vi "LS-50.vi"(0 "LS-50 Notifier":refnum<notifier>, 5 "LS-50 Action":T1={"Action"=enum."Get Position", "Axis"=[], "Setpoint"=[], "Velocity"=0.5, "Cmd Recvd?"=FALSE, "Position"=[], "Status"=enum."Error", "Misc"=variant} {"Velocity" min=0.0 max=1.0 step=0.01}, 11 "LS-50 VISA":refnum<visa-resource-name>) -> (4 "LS-50 Notifier (Dup)":refnum<notifier>)   [LabVIEW 2020]
uses:
  Stages Controls/Stage Notifier Element.ctl
  Stages Controls/Stage Actions.ctl
  Stages Controls/Stage Status.ctl
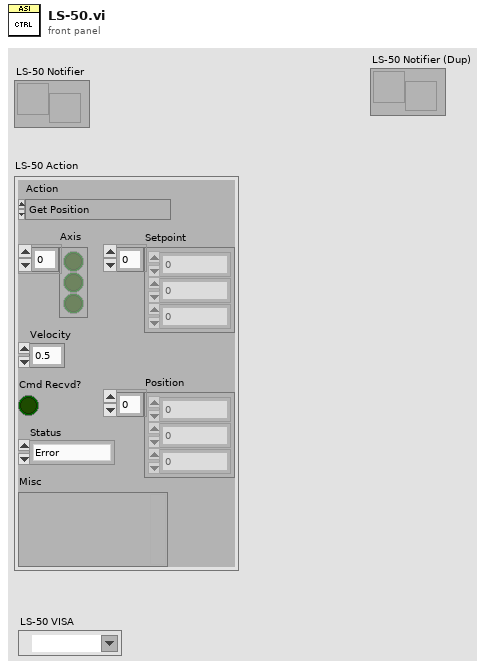
[diagram p1: front panel]
types:
  T1 = typedef "Stage Notifier Element.ctl" = cluster{"Action":T2, "Axis":bool[], "Setpoint":dbl[], "Velocity":dbl, "Cmd Recvd?":bool, "Position":dbl[], "Status":T3, "Misc":variant}
  T2 = typedef "Stage Actions.ctl" = enum16{"Get Position", "MVR", "MOVE", "HALT", "ONTARGET", "ERROR", "REFERENCE", "INIT", "VELOCITY", "STATUS", "EXIT", "HOME", "ZEROPOS", "NANOPOS", "ANALOG", "QUIT"}
  T3 = typedef "Stage Status.ctl" = enum16{"Error", "Abort", "Busy", "On Target"}
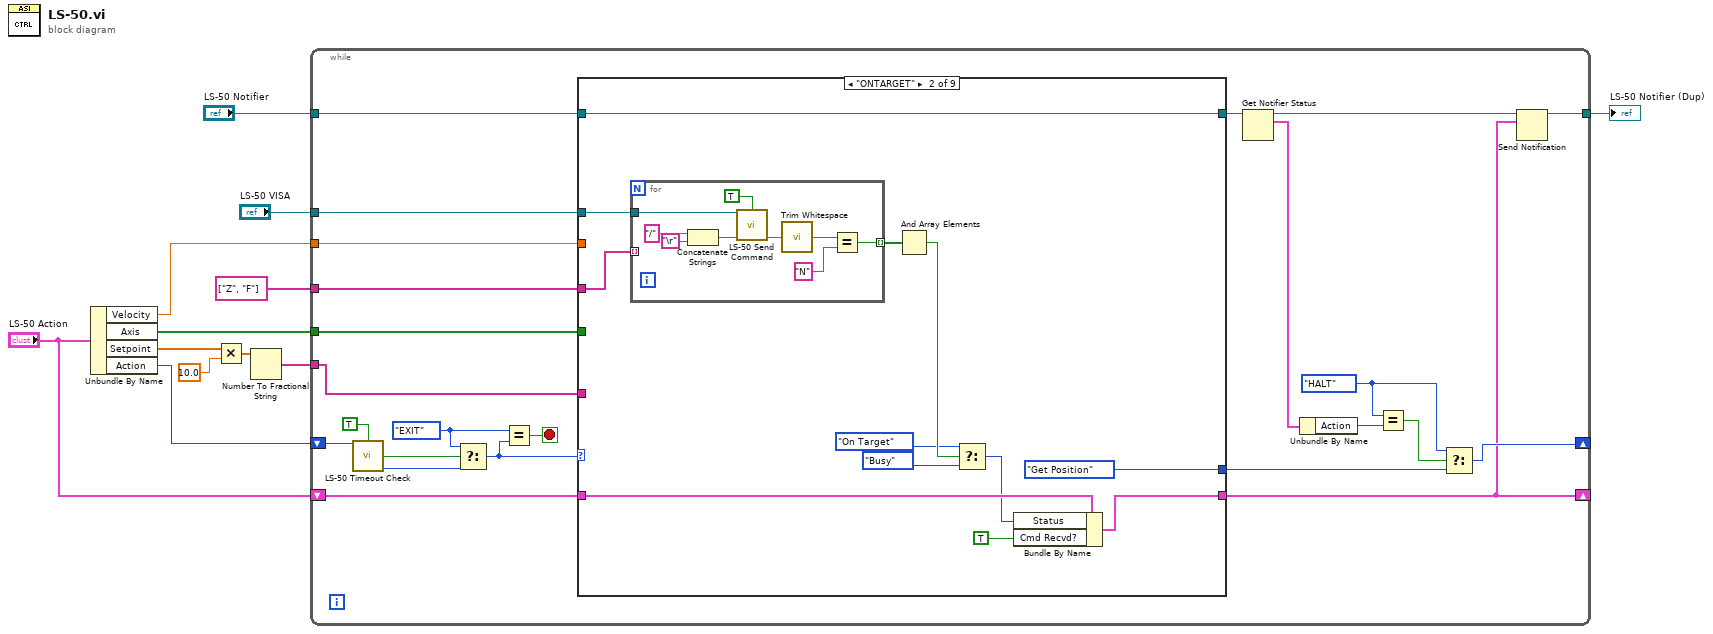
[diagram p0: block diagram]
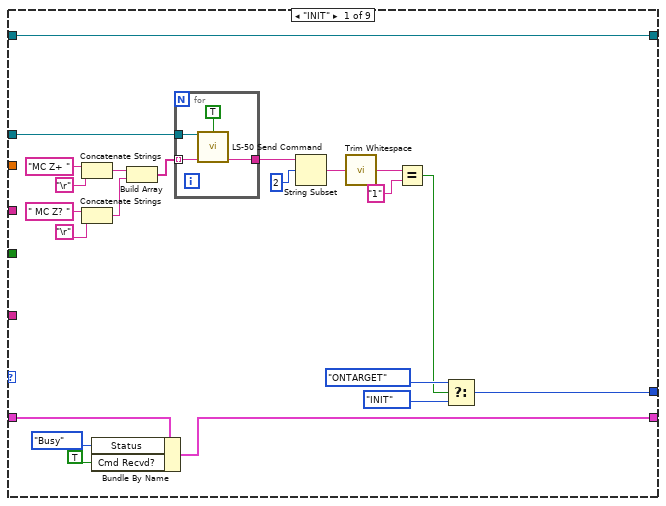
[diagram p2: hidden frame]
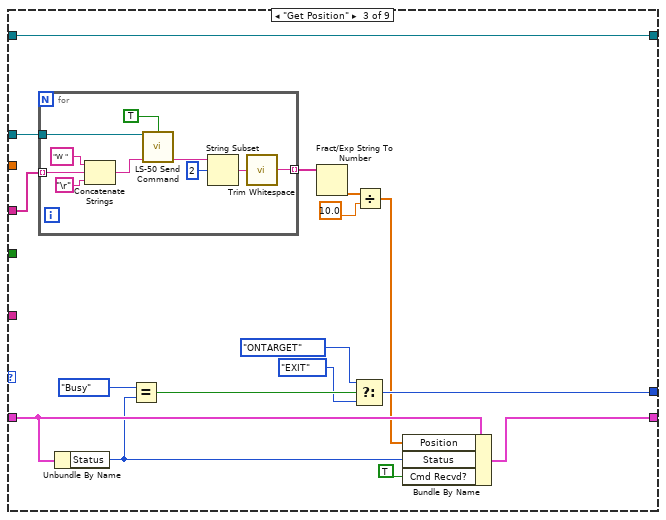
[diagram p3: hidden frame]
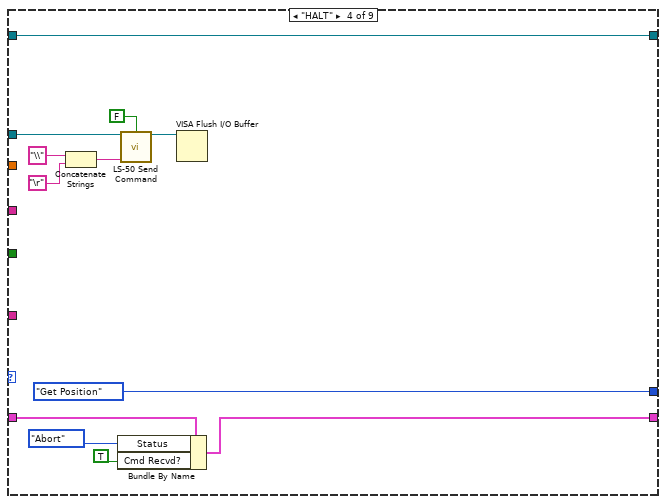
[diagram p4: hidden frame]
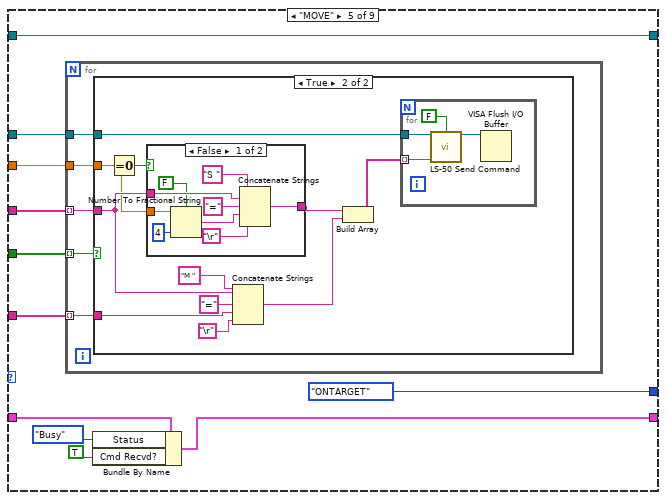
[diagram p5: hidden frame]
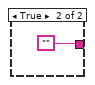
[diagram p7: hidden frame]
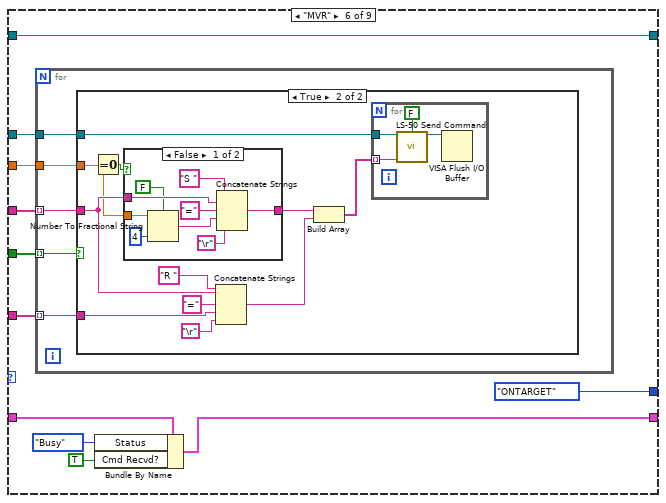
[diagram p8: hidden frame]
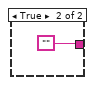
[diagram p10: hidden frame]
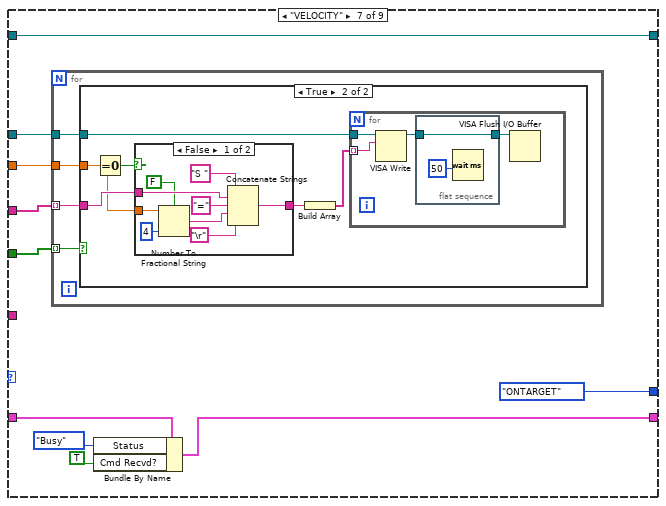
[diagram p11: hidden frame]
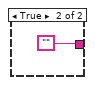
[diagram p13: hidden frame]
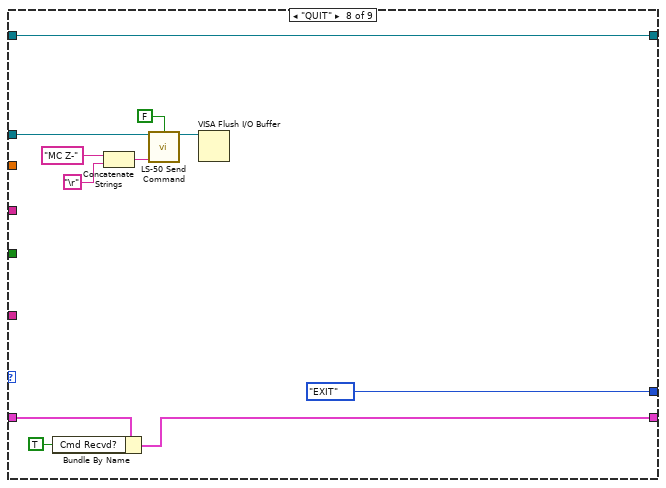
[diagram p14: hidden frame]
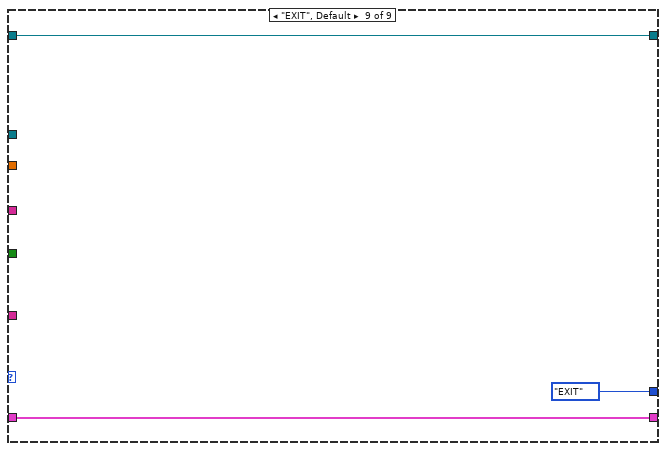
[diagram p15: hidden frame]
diagram:
  n1 = Unbundle By Name("LS-50 Action") -> ("Velocity"=w9:dbl, "Axis"=w8:bool[], "Setpoint"=w5:dbl[], "Action"=w7:T2)
  n2 = Multiply(x=w5, y=10.0) -> (x*y=w6:dbl[])
  n3 = Number To Fractional String(number=w6) -> (F-format string=w10:string[])  [unwired: 3 in]
  n4 = while {
    tunnel: string[] ["Z", "F"] -> [w36]
    shift-right: [w28] -> _
    shift-left: w7 -> [w25]
    tunnel: w8 -> [w33]
    tunnel: w9 -> [w32]
    tunnel: w10 -> [w34]
    shift-right: [w27] -> _
    shift-left: "LS-50 Action" -> [w30]
    tunnel: "LS-50 VISA" -> [w35]
    tunnel: "LS-50 Notifier" -> [w15]
    tunnel: [w13] -> w1
    stop <- w31 stop-if-true
    w17 = Stage_Actions."HALT" ("Action")
    w22 = Stage_Actions."EXIT" ("t")
    n5 = call "LS-50 Timeout Check.vi"("Action"=w25, "User Input?"=TRUE) -> ("Timeout?"=w24:bool, "Action (Dup)"=w23:T2)  [unwired: 12 in]
    n6 = Select(t=w22, s=w24, f=w23) -> (s? t:f=w21:T2)
    n7 = Equal?(x=w22, y=w21) -> (x = y?=w31:bool)
    n8 = case shown="\"ONTARGET\"" w21 {
      tunnel: w36 -> [_ w73 w99 _ w132 w173 w213 _ _]
      tunnel: w35 -> [w40 w64 w85 w114 w123 w164 w205 w244 _]
      tunnel: w34 -> [_ _ _ _ w131 w172 _ _ _]
      tunnel: w33 -> [_ _ _ _ w130 w171 w212 _ _]
      tunnel: w32 -> [_ _ _ _ w129 w170 w211 _ _]
      tunnel: [w50 Stage_Actions."Get Position" ("y") w95 Stage_Actions."Get Position" ("Action") Stage_Actions."ONTARGET" ("y") Stage_Actions."ONTARGET" ("y") Stage_Actions."ONTARGET" ("y") Stage_Actions."EXIT" ("y") Stage_Actions."EXIT" ("y")] -> w29
      tunnel: w30 -> [w47 w70 w90 w116 w128 w166 w207 w246 w253]
      tunnel: [w46 w71 w89 w117 w125 w167 w208 w245 w253] -> w27
      tunnel: [w37 w63 w84 w110 w122 w163 w204 w240 w251] -> w14
      tunnel: w15 -> [w37 w63 w84 w110 w122 w163 w204 w240 w251]
      frame "INIT" {
        n9 = Concatenate Strings("MC Z+ " ("string"), "\r") -> (w43:string)
        n10 = Concatenate Strings(" MC Z? " ("string"), "\r") -> (w42:string)
        n11 = Bundle By Name(cluster=w47, "Status"=Stage_Status."Busy", "Cmd Recvd?"=TRUE) -> (w46:T1)
        n12 = Build Array(w43, w42) -> (w41:string[])
        n13 = for {
          tunnel: [w60] -> w39
          tunnel: w41 -> [w61] mode=indexing
          tunnel: w40 -> [w62]
          n14 = call "LS-50 Send Command.vi"("VISA Ref"=w62, "Read Reply?"=TRUE, "Command"=w61) -> ("Response"=w60:string)  [unwired: 10 in, 2 out]
        }
        n15 = String Subset(string=w39, offset (0)=2) -> (substring=w56:string)  [unwired: 1 in]
        n16 = call <vilib>:"Trim Whitespace.vi"("string"=w56) -> ("trimmed string"=w57:string)  [unwired: 1 in]
        n17 = Equal?(x=w57, y="1") -> (x = y?=w38:bool)
        n18 = Select(t=Stage_Actions."ONTARGET" ("y"), s=w38, f=Stage_Actions."INIT" ("y")) -> (s? t:f=w50:T2)
      }
      frame "ONTARGET" {
        n19 = for {
          tunnel: [w83] -> w74 mode=indexing
          tunnel: w73 -> [_] mode=indexing
          tunnel: w64 -> [w78]
          n20 = Concatenate Strings("/" ("string"), "\r") -> (w77:string)
          n21 = call "LS-50 Send Command.vi"("VISA Ref"=w78, "Read Reply?"=TRUE ("Wait for Reply?"), "Command"=w77) -> ("Response"=w76:string)  [unwired: 10 in, 2 out]
          n22 = call <vilib>:"Trim Whitespace.vi"("string"=w76) -> ("trimmed string"=w80:string)  [unwired: 1 in]
          n23 = Equal?(x=w80, y="N") -> (x = y?=w83:bool)
        }
        n24 = And Array Elements(Boolean array=w74) -> (logical AND=w68:bool)
        n25 = Select(t=Stage_Status."On Target" ("Status"), s=w68, f=Stage_Status."Busy" ("Status")) -> (s? t:f=w66:T3)
        n26 = Bundle By Name(cluster=w70, "Status"=w66, "Cmd Recvd?"=TRUE) -> (w71:T1)
      }
      frame "Get Position" {
        n27 = for {
          tunnel: [w109] -> w98 mode=indexing
          tunnel: w99 -> [w104] mode=indexing
          tunnel: w85 -> [w103]
          n28 = Concatenate Strings("W " ("string"), w104, "\r") -> (w102:string)
          n29 = call "LS-50 Send Command.vi"("VISA Ref"=w103, "Read Reply?"=TRUE ("Wait for Reply?"), "Command"=w102) -> ("Response"=w101:string)  [unwired: 10 in, 2 out]
          n30 = String Subset(string=w101, offset (0)=2) -> (substring=w105:string)  [unwired: 1 in]
          n31 = call <vilib>:"Trim Whitespace.vi"("string"=w105) -> ("trimmed string"=w109:string)  [unwired: 1 in]
        }
        n32 = Unbundle By Name(w90) -> ("Status"=w87:T3)
        n33 = Equal?(x=Stage_Status."Busy", y=w87) -> (x = y?=w93:bool)
        n34 = Fract/Exp String To Number(string=w98) -> (number=w96:dbl[])  [unwired: 3 in, 1 out]
        n35 = Select(t=Stage_Actions."ONTARGET" ("Action"), s=w93, f=Stage_Actions."EXIT" ("Action")) -> (s? t:f=w95:T2)
        n36 = Divide(x=w96, y=10.0) -> (x/y=w88:dbl[])
        n37 = Bundle By Name(cluster=w90, "Position"=w88, "Status"=w87, "Cmd Recvd?"=TRUE) -> (w89:T1)
      }
      frame "HALT" {
        n38 = Concatenate Strings("\\" ("string"), "\r") -> (w112:string)
        n39 = Bundle By Name(cluster=w116, "Status"=Stage_Status."Abort", "Cmd Recvd?"=TRUE) -> (w117:T1)
        n40 = call "LS-50 Send Command.vi"("VISA Ref"=w114, "Read Reply?"=FALSE, "Command"=w112) -> ("VISA Ref Out"=w113:refnum<visa-resource-name>)  [unwired: 10 in, 2 out]
        n41 = VISA Flush I/O Buffer(VISA resource name=w113) -> ()  [unwired: 2 in, 2 out]
      }
      frame "MOVE" {
        n42 = for {
          tunnel: w132 -> [w137] mode=indexing
          tunnel: w131 -> [w136] mode=indexing
          tunnel: w130 -> [w135] mode=indexing
          tunnel: w129 -> [w134]
          tunnel: w123 -> [w133]
          n43 = case shown="True" w135 {
            tunnel: w137 -> [_ w144]
            tunnel: w136 -> [_ w145]
            tunnel: w133 -> [_ w138]
            tunnel: w134 -> [_ w143]
            frame False {
            }
            frame True {
              n44 = Equal To 0?(x=w143) -> (x = 0?=w142:bool)
              n45 = case shown="False" w142 {
                tunnel: w144 -> [w158 _]
                tunnel: w143 -> [w155 _]
                tunnel: [w157 ""] -> w141
                frame False {
                  n46 = Number To Fractional String(use system decimal point (T)=FALSE, number=w155, precision (6)=i16 4) -> (F-format string=w156:string)  [unwired: 1 in]
                  n47 = Concatenate Strings("S ", w158, "=", w156, "\r") -> (w157:string)
                }
                frame True {
                }
              }
              n48 = Concatenate Strings("M ", w144, "=", w145, "\r") -> (w140:string)
              n49 = Build Array(w141, w140) -> (w139:string[])
              n50 = for {
                tunnel: w139 -> [w150] mode=indexing
                tunnel: w138 -> [w152]
                n51 = call "LS-50 Send Command.vi"("VISA Ref"=w152, "Read Reply?"=FALSE, "Command"=w150) -> ("VISA Ref Out"=w151:refnum<visa-resource-name>)  [unwired: 10 in, 2 out]
                n52 = VISA Flush I/O Buffer(VISA resource name=w151) -> ()  [unwired: 2 in, 2 out]
              }
            }
          }
        }
        n53 = Bundle By Name(cluster=w128, "Status"=Stage_Status."Busy", "Cmd Recvd?"=TRUE) -> (w125:T1)
      }
      frame "MVR" {
        n54 = for {
          tunnel: w173 -> [w178] mode=indexing
          tunnel: w172 -> [w177] mode=indexing
          tunnel: w171 -> [w176] mode=indexing
          tunnel: w170 -> [w175]
          tunnel: w164 -> [w174]
          n55 = case shown="True" w176 {
            tunnel: w178 -> [_ w185]
            tunnel: w177 -> [_ w186]
            tunnel: w174 -> [_ w179]
            tunnel: w175 -> [_ w184]
            frame False {
            }
            frame True {
              n56 = Equal To 0?(x=w184) -> (x = 0?=w183:bool)
              n57 = case shown="False" w183 {
                tunnel: w185 -> [w199 _]
                tunnel: w184 -> [w197 _]
                tunnel: [w198 ""] -> w182
                frame False {
                  n58 = Number To Fractional String(use system decimal point (T)=FALSE, number=w197, precision (6)=i16 4) -> (F-format string=w196:string)  [unwired: 1 in]
                  n59 = Concatenate Strings("S ", w199, "=", w196, "\r") -> (w198:string)
                }
                frame True {
                }
              }
              n60 = Concatenate Strings("R ", w185, "=", w186, "\r") -> (w181:string)
              n61 = Build Array(w182, w181) -> (w180:string[])
              n62 = for {
                tunnel: w180 -> [w192] mode=indexing
                tunnel: w179 -> [w193]
                n63 = call "LS-50 Send Command.vi"("VISA Ref"=w193, "Read Reply?"=FALSE, "Command"=w192) -> ("VISA Ref Out"=w191:refnum<visa-resource-name>)  [unwired: 10 in, 2 out]
                n64 = VISA Flush I/O Buffer(VISA resource name=w191) -> ()  [unwired: 2 in, 2 out]
              }
            }
          }
        }
        n65 = Bundle By Name(cluster=w166, "Status"=Stage_Status."Busy", "Cmd Recvd?"=TRUE) -> (w167:T1)
      }
      frame "VELOCITY" {
        n66 = for {
          tunnel: w213 -> [w217] mode=indexing
          tunnel: w212 -> [w216] mode=indexing
          tunnel: w211 -> [w215]
          tunnel: w205 -> [w214]
          n67 = case shown="True" w216 {
            tunnel: w217 -> [_ w223]
            tunnel: w214 -> [_ w218]
            tunnel: w215 -> [_ w222]
            frame False {
            }
            frame True {
              n68 = Equal To 0?(x=w222) -> (x = 0?=w221:bool)
              n69 = case shown="False" w221 {
                tunnel: w223 -> [w235 _]
                tunnel: w222 -> [w232 _]
                tunnel: [w234 ""] -> w220
                frame False {
                  n70 = Number To Fractional String(use system decimal point (T)=FALSE, number=w232, precision (6)=i16 4) -> (F-format string=w233:string)  [unwired: 1 in]
                  n71 = Concatenate Strings("S ", w235, "=", w233, "\r") -> (w234:string)
                }
                frame True {
                }
              }
              n72 = Build Array(w220) -> (w219:string[])
              n73 = for {
                tunnel: w219 -> [w227] mode=indexing
                tunnel: w218 -> [w224]
                n74 = VISA Write(VISA resource name=w224, write buffer=w227) -> (VISA resource name out=w226:refnum<visa-resource-name>)  [unwired: 1 in, 2 out]
                n75 = flat-sequence {
                  tunnel: [w228] -> w225
                  tunnel: w226 -> [w228]
                  frame #0 {
                    n76 = Wait (ms)(milliseconds to wait=u32 50) -> ()  [unwired: 1 out]
                  }
                }
                n77 = VISA Flush I/O Buffer(VISA resource name=w225) -> ()  [unwired: 2 in, 2 out]
              }
            }
          }
        }
        n78 = Bundle By Name(cluster=w207, "Status"=Stage_Status."Busy", "Cmd Recvd?"=TRUE) -> (w208:T1)
      }
      frame "QUIT" {
        n79 = Bundle By Name(cluster=w246, "Cmd Recvd?"=TRUE) -> (w245:T1)
        n80 = Concatenate Strings("MC Z-" ("write buffer"), "\r") -> (w243:string)
        n81 = call "LS-50 Send Command.vi"("VISA Ref"=w244, "Read Reply?"=FALSE, "Command"=w243) -> ("VISA Ref Out"=w242:refnum<visa-resource-name>)  [unwired: 10 in, 2 out]
        n82 = VISA Flush I/O Buffer(VISA resource name=w242) -> ()  [unwired: 2 in, 2 out]
      }
      frame "EXIT", Default {
      }
    }
    n83 = Get Notifier Status(notifier=w14) -> (notifier out=w20:refnum<notifier>, current notification=w16:T1)  [unwired: 1 in, 3 out]
    n84 = Unbundle By Name(w16) -> ("Action"=w18:T2)
    n85 = Equal?(x=w17, y=w18) -> (x = y?=w19:bool)
    n86 = Select(t=w17, s=w19, f=w29) -> (s? t:f=w28:T2)
    n87 = Send Notification(notification=w27, notifier=w20) -> (notifier out=w13:refnum<notifier>)  [unwired: 1 in, 1 out]
  }
  "LS-50 Notifier (Dup)" <- w1
